vi "create_filename.vi"() -> ()   [LabVIEW 2018]
panel:
  out "appended path":path
  in  "path":path
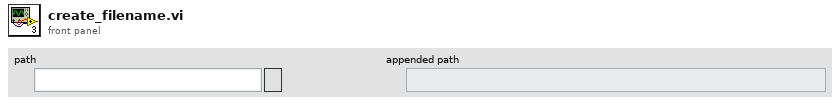
[diagram p1: front panel]
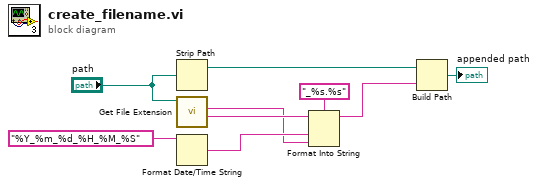
[diagram p0: block diagram]
diagram:
  n1 = Strip Path(path="path") -> (stripped path=w9:path)  [unwired: 1 out]
  n2 = call <vilib>:"Get File Extension.vi"("file"="path") -> ("filename without extension"=w8:string, "lowercase file extension"=w5:string)  [unwired: 6 in, 3 out]
  n3 = Format Date/Time String(time format string (%c)="%Y_%m_%d_%H_%M_%S") -> (date/time string=w6:string)  [unwired: 2 in]
  n4 = Format Into String(format string="_%s.%s", initial string=w8, w6, w5) -> (resulting string=w4:string)  [unwired: 1 in, 1 out]
  n5 = Build Path(base path=w9, name or relative path=w4) -> (appended path=→"appended path":path)
